vi "InitCmdLib.vi"(8 "error in (no error)":errorcluster, 11 "logging":bool) -> (0 "error out":errorcluster, 2 "Device Key":string, 3 "CmdLib":refnum<k24>)   [LabVIEW 2021]
uses:
  C:/_git/mantoles-dev-box/LabVIEW/sample-code/LabVIEW 2010/PowerMeterCommands.dll
  PowerMeterCommands.dll
panel:
  in  "deviceKey":string
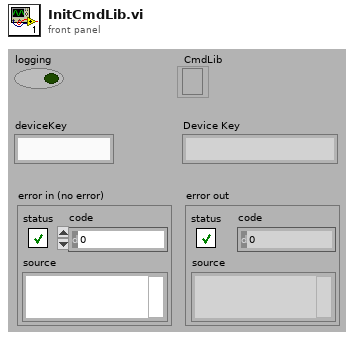
[diagram p1: front panel]
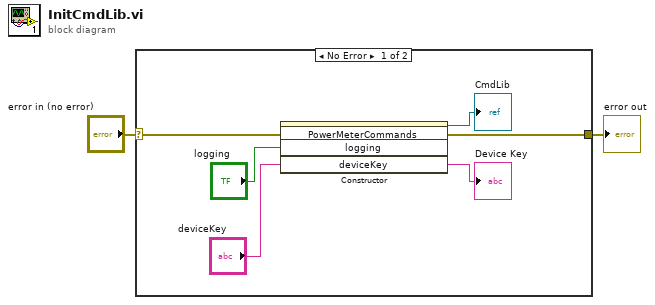
[diagram p0: block diagram]
diagram:
  n1 = case shown="No Error" "error in (no error)" {
    selector: "error in (no error)" -> [w5 w9]
    tunnel: [w4 w9] -> w1
    frame No Error {
      n2 = constructor class="PowerMeterCommands"(error in=w5, "logging"="logging", "deviceKey"="deviceKey") -> (reference out=→"CmdLib":refnum<k24>, error out=w4:errorcluster, "deviceKey"=→"Device Key":string)  [unwired: 2 in, 2 out]
    }
    frame Error {
    }
  }
  "error out" <- w1
